vi "CAPTH-Analysis Thread.vi"(0 "Params":T2={"Stimulus"={"EAR"=enum."RIGHT", "HI FREQ"=18.0, "LO FREQ"=5.0, "FREQ STEP"=8, "Rep Rate (/s)"=20.0, "Alternate Polarity"=TRUE, "# CYCLES"=1, "Duration (ms)"=0.0, "Ramp (ms)"=0.0}, "Response"={"Averages (3dB steps)"=12, "Time Window (ms)"=8.5, "dt (us)"=10.0, "Grass gain"=1000.0, "CRITERION (mV)"=60.0, "CEILING (dB atten)"=6.0, "Use previous"=FALSE, "Save avgs"=FALSE, "Save raw"=FALSE, "Save history"=FALSE, "CEILING (dB SPL)"=6.0}} {"Response"."CRITERION (mV)" format="%.2f"; "Response"."Time Window (ms)" format="%.2f"}, 5 "Datafile":path, 7 "IPC":T1, 9 "avg refs":refnum<vi>[](array[refnum])) -> (15 "error out":errorcluster)   [LabVIEW 2020]
uses:
  Typedefs/CAPTH-Parameters.ctl
  Typedefs/CAPTH-Stimulus.ctl
  Typedefs/CAPTH-Response.ctl
  Typedefs/CAPTH-IPC.ctl
  Typedefs/CAPTH-Start Data.ctl
  Typedefs/CAPTH-Analysis Message.ctl
  Typedefs/CAPTH-Analysis Action.ctl
  Typedefs/CAPTH-StimCon.ctl
  Typedefs/CAPTH-Analysis Data Properties.ctl
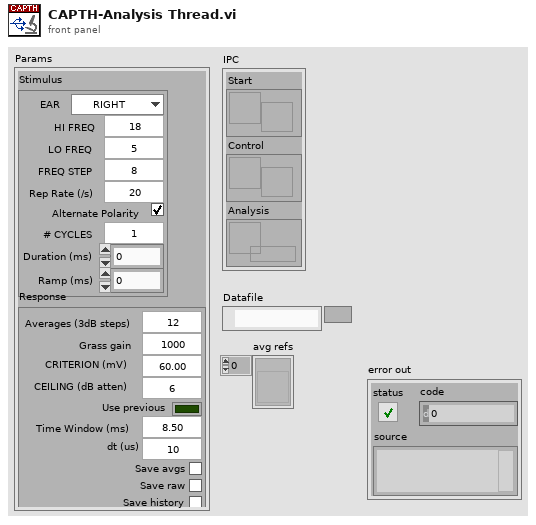
[diagram p1: front panel]
types:
  T1 = typedef "CAPTH-IPC.ctl" = cluster{"Start":refnum<notifier>, "Control":refnum<notifier>, "Analysis":refnum<queue>}
  T2 = typedef "CAPTH-Parameters.ctl" = cluster{"Stimulus":T3, "Response":T4}
  T3 = typedef "CAPTH-Stimulus.ctl" = cluster{"EAR":enum16{"RIGHT", "LEFT\n", "ALTERNATE"}, "HI FREQ":dbl, "LO FREQ":dbl, "FREQ STEP":u8, "Rep Rate (/s)":dbl, "Alternate Polarity":bool, "# CYCLES":u8, "Duration (ms)":dbl, "Ramp (ms)":dbl}
  T4 = typedef "CAPTH-Response.ctl" = cluster{"Averages (3dB steps)":i32, "Time Window (ms)":dbl, "dt (us)":dbl, "Grass gain":dbl, "CRITERION (mV)":dbl, "CEILING (dB atten)":dbl, "Use previous":bool, "Save avgs":bool, "Save raw":bool, "Save history":bool, "CEILING (dB SPL)":dbl}
  T5 = typedef "CAPTH-Analysis State.ctl" = cluster{"History":T6, "Freq":dbl[], "StimCon":T7, "datafile":path, "raw":refnum<file>, "avg":refnum<file>}
  T6 = typedef "CAPTH-History.ctl" = cluster{"MaxSPL":dbl, "atten":dbl[], "Vp-p":dbl[], "Ntries":i32[]}[][]
  T7 = typedef "CAPTH-StimCon.ctl" = cluster{"ear":i32, "freq":i32, "Max SPL":dbl}
  T8 = typedef "CAPTH-Analysis Message.ctl" = cluster{"Action":T9, "Data":dbl[], "StimCon":T7, "Properties":T10, "Num":i32}
  T9 = typedef "CAPTH-Analysis Action.ctl" = enum16{"Init", "Raw", "Avg", "Quit"}
  T10 = typedef "CAPTH-Analysis Data Properties.ctl" = cluster{"atten":dbl, "amp":dbl, "1dB":bool}
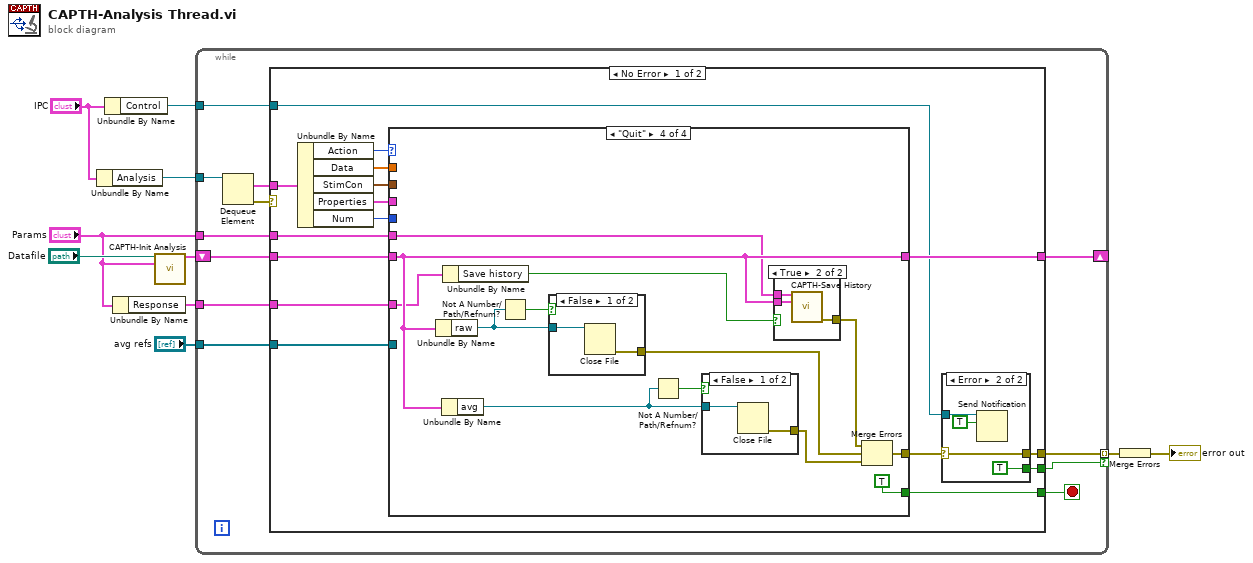
[diagram p0: block diagram]
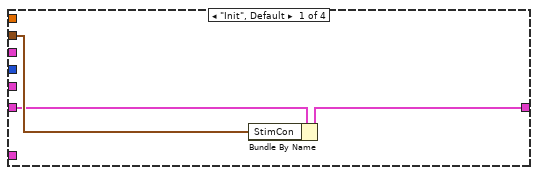
[diagram p3: hidden frame]
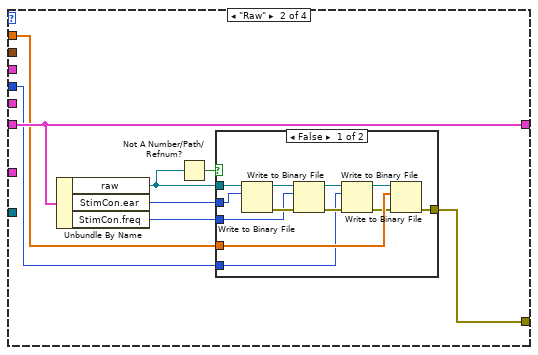
[diagram p4: hidden frame]
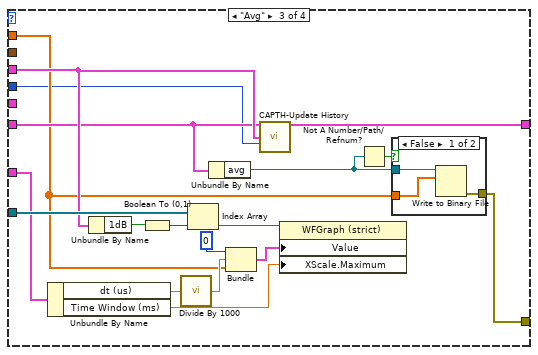
[diagram p6: hidden frame]
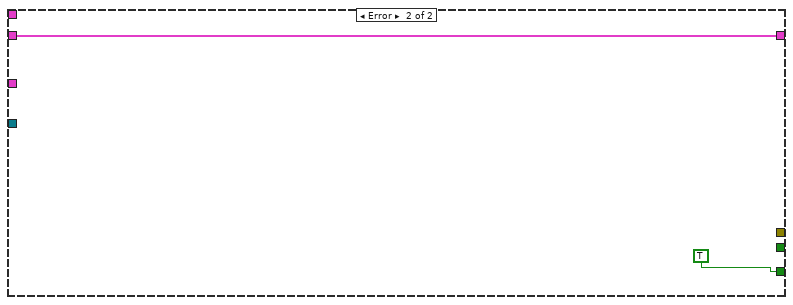
[diagram p11: hidden frame]
diagram:
  n1 = Unbundle By Name("IPC") -> ("Analysis"=w10:refnum<queue>)
  n2 = Unbundle By Name("IPC") -> ("Control"=w3:refnum<notifier>)
  n3 = Unbundle By Name("Params") -> ("Response"=w6:T4)
  n4 = call "CAPTH-Init Analysis.vi"("Datafile"="Datafile", "Params"="Params") -> ("State"=w8:T5)  [unwired: 12 in, 1 out]
  n5 = while {
    tunnel: w10 -> [w22]
    tunnel: "avg refs" -> [w18]
    shift-right: [w15] -> _
    shift-left: w8 -> [w16]
    tunnel: w6 -> [w17]
    tunnel: "Params" -> [w14]
    tunnel: w3 -> [w13]
    tunnel: [w12] -> w2 mode=indexing if=w11
    stop <- w19 stop-if-true
    n6 = Dequeue Element(queue=w22) -> (element=w20:T8, error out=w21:errorcluster)  [unwired: 2 in, 2 out]
    n7 = case shown="No Error" w21 {
      tunnel: w20 -> [w38 _]
      tunnel: [w36 TRUE] -> w19
      tunnel: w18 -> [w32 _]
      tunnel: w17 -> [w31 _]
      tunnel: w16 -> [w30 w108]
      tunnel: [w29 w108] -> w15
      tunnel: [w26 _] -> w12
      tunnel: w14 -> [w28 _]
      tunnel: w13 -> [w25 _]
      tunnel: [w24 _] -> w11
      frame No Error {
        n8 = Unbundle By Name(w38) -> ("Action"=w37:T9, "Data"=w35:dbl[], "StimCon"=w34:T7, "Properties"=w33:T10, "Num"=w23:i32)
        n9 = case shown="\"Quit\"" w37 {
          tunnel: [_ _ _ TRUE] -> w36
          tunnel: w35 -> [_ w49 w71 _]
          tunnel: w34 -> [w45 _ _ _]
          tunnel: w33 -> [_ _ w73 _]
          tunnel: w32 -> [_ _ w83 _]
          tunnel: w31 -> [_ _ w77 w89]
          tunnel: w30 -> [w44 w54 w72 w92]
          tunnel: [w46 w54 w74 w92] -> w29
          tunnel: [_ w48 w68 w97] -> w27
          tunnel: w28 -> [_ _ _ w90]
          tunnel: w23 -> [_ w47 w67 _]
          frame "Init", Default {
            n10 = Bundle By Name(cluster=w44, "StimCon"=w45) -> (w46:T5)
          }
          frame "Raw" {
            n11 = Unbundle By Name(w54) -> ("raw"=w52:refnum<file>, "StimCon.ear"=w51:i32, "StimCon.freq"=w50:i32)
            n12 = Not A Number/Path/Refnum?(number/path/refnum=w52) -> (NaN/Path/Refnum?=w53:bool)
            n13 = case shown="False" w53 {
              tunnel: w52 -> [w66 _]
              tunnel: w51 -> [w65 _]
              tunnel: w50 -> [w62 _]
              tunnel: w49 -> [w61 _]
              tunnel: [w60 _] -> w48
              tunnel: w47 -> [w55 _]
              frame False {
                n14 = Write to Binary File(file (use dialog)=w66, data=w65) -> (refnum out=w64:refnum<file>, error out=w63:errorcluster)  [unwired: 4 in, 1 out]
                n15 = Write to Binary File(file (use dialog)=w64, data=w62, error in=w63) -> (refnum out=w56:refnum<file>, error out=w59:errorcluster)  [unwired: 3 in, 1 out]
                n16 = Write to Binary File(file (use dialog)=w56, data=w55, error in=w59) -> (refnum out=w57:refnum<file>, error out=w58:errorcluster)  [unwired: 3 in, 1 out]
                n17 = Write to Binary File(file (use dialog)=w57, data=w61, error in=w58) -> (error out=w60:errorcluster)  [unwired: 3 in, 2 out]
              }
              frame True {
              }
            }
          }
          frame "Avg" {
            n18 = Unbundle By Name(w77) -> ("dt (us)"=w78:dbl, "Time Window (ms)"=w75:dbl)
            n19 = Unbundle By Name(w73) -> ("1dB"=w84:bool)
            n20 = Boolean To (0,1)(Boolean=w84) -> (0, 1=w82:i16)
            n21 = call "Divide By 1000.vi"("X"=w78) -> ("X/1000"=w76:dbl)
            n22 = Index Array(array=w83, index=w82) -> (element=w79:refnum<vi>)
            n23 = Unbundle By Name(w72) -> ("avg"=w69:refnum<file>)
            n24 = Bundle(0, "X/1000"=w76, "Data"=w71) -> (w81:cluster{i32, "X/1000":dbl, "Data":dbl[]})  [unwired: 1 in]
            n25 = call "CAPTH-Update History.vi"("State in"=w72, "Properties"=w73, "Ntries"=w67) -> ("State out"=w74:T5)  [unwired: 12 in]
            n26 = property class="WFGraph (strict)"(reference=w79, "Value"=w81, "XScale.Maximum"=w75) -> ()  [unwired: 1 in, 2 out]
            n27 = Not A Number/Path/Refnum?(number/path/refnum=w69) -> (NaN/Path/Refnum?=w70:bool)
            n28 = case shown="False" w70 {
              tunnel: [w87 _] -> w68
              tunnel: w69 -> [w86 _]
              tunnel: w71 -> [w85 _]
              frame False {
                n29 = Write to Binary File(file (use dialog)=w86, data=w85) -> (error out=w87:errorcluster)  [unwired: 4 in, 2 out]
              }
              frame True {
              }
            }
          }
          frame "Quit" {
            n30 = Unbundle By Name(w92) -> ("raw"=w99:refnum<file>)
            n31 = Unbundle By Name(w92) -> ("avg"=w98:refnum<file>)
            n32 = Unbundle By Name(w89) -> ("Save history"=w88:bool)
            n33 = Not A Number/Path/Refnum?(number/path/refnum=w99) -> (NaN/Path/Refnum?=w94:bool)
            n34 = case shown="False" w94 {
              tunnel: w99 -> [w107 _]
              tunnel: [w106 _] -> w95
              frame False {
                n35 = Close File(refnum=w107) -> (error out=w106:errorcluster)  [unwired: 1 in, 1 out]
              }
              frame True {
              }
            }
            n36 = Not A Number/Path/Refnum?(number/path/refnum=w98) -> (NaN/Path/Refnum?=w93:bool)
            n37 = case shown="False" w93 {
              tunnel: w98 -> [w105 _]
              tunnel: [w104 _] -> w96
              frame False {
                n38 = Close File(refnum=w105) -> (error out=w104:errorcluster)  [unwired: 1 in, 1 out]
              }
              frame True {
              }
            }
            n39 = case shown="True" w88 {
              tunnel: w92 -> [_ w103]
              tunnel: [_ w102] -> w91
              tunnel: w90 -> [_ w101]
              frame False {
              }
              frame True {
                n40 = call "CAPTH-Save History.vi"("Params"=w101, "State"=w103) -> ("error out"=w102:errorcluster)  [unwired: 13 in]
              }
            }
            n41 = Merge Errors(w91, w95, w96) -> (w97:errorcluster)
          }
        }
        n42 = case shown="Error" w27 {
          selector: w27 -> [w39 w43]
          tunnel: [w39 w43] -> w26
          tunnel: w25 -> [_ w42]
          tunnel: [_ TRUE] -> w24
          frame No Error {
          }
          frame Error {
            n43 = Send Notification(notification=TRUE, notifier=w42) -> ()  [unwired: 1 in, 2 out]
          }
        }
      }
      frame Error {
      }
    }
  }
  n44 = Merge Errors(w2) -> (→"error out":errorcluster)
